vi "Hardware-LEDs-Flash.vi"(5 "Period (s)":sgl, 7 "dt (s)":sgl, 11 "Reset":bool) -> (0 "Count":u32, 3 "Output":bool)   [LabVIEW 2016, in "DSI-RT.lvlib"]
uses:
  DSI-RT.lvlib
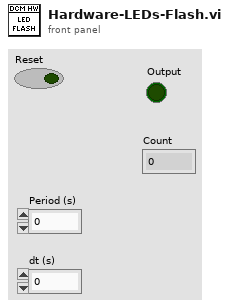
[diagram p1: front panel]
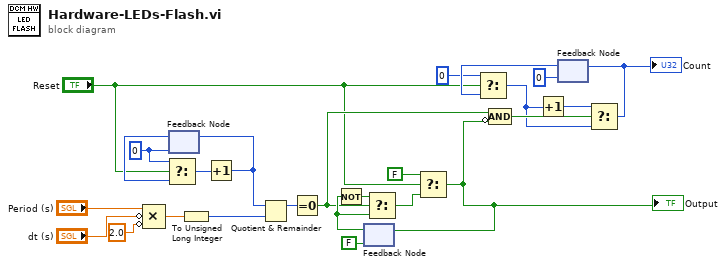
[diagram p0: block diagram]
diagram:
  w16 = u32 0
  n1 = Compound Arithmetic op=MULTIPLY("Period (s)", invert "dt (s)", invert sgl 2.0 ("value")) -> (w17:sgl)
  n2 = feedback #1(w16) -> (w7:u32)
  n3 = Select(t=w16, s="Reset", f=w7) -> (s? t:f=w6:u32)
  n4 = To Unsigned Long Integer(number=w17) -> (unsigned 32bit integer=w21:u32)
  n5 = Increment(x=w6) -> (x+1=w5:u32)
  n6 = feedback-in #1(w5) -> ()
  n7 = Quotient & Remainder(x=w5, y=w21) -> (x-y*floor(x/y)=w22:u32)  [unwired: 1 out]
  n8 = Equal To 0?(x=w22) -> (x = 0?=w13:bool)
  n9 = feedback #2(FALSE) -> (w18:bool)
  n10 = Not(x=w18) -> (.not. x?=w19:bool)
  n11 = Select(t=w19, s=w13, f=w18) -> (s? t:f=w4:bool)
  n12 = Select(t=FALSE, s="Reset", f=w4) -> (s? t:f=w3:bool)
  "Output" <- w3
  n13 = feedback-in #2(w3) -> ()
  n14 = Compound Arithmetic op=AND(w13, invert w3) -> (w12:bool)
  n15 = feedback #3(u32 0) -> (w10:u32)
  n16 = Select(t=u32 0, s="Reset", f=w10) -> (s? t:f=w9:u32)
  n17 = Increment(x=w9) -> (x+1=w15:u32)
  n18 = Select(t=w15, s=w12, f=w9) -> (s? t:f=w11:u32)
  "Count" <- w11
  n19 = feedback-in #3(w11) -> ()
